vi "CreateGraphMenu_InAreaButNotCurve.vi"(4 "isFloatXY":T1, 6 "isShowYvalue":T1, 9 "Language":refnum<vi>, 11 "菜单输入":refnum<k9>) -> ()   [LabVIEW 2015]
uses:
  Ctrls/YesOrNo.ctl
  GlobalVariables.vi
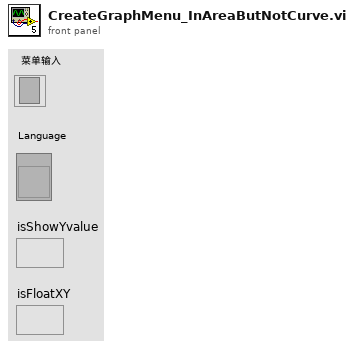
[diagram p1: front panel]
types:
  T1 = typedef "YesOrNo.ctl" = bool
  T2 = cluster{"MenuNames":string[], "MenuTags":string[]}
  T3 = cluster{"Visible":bool, "Color":u32, "LineWidth":u8}
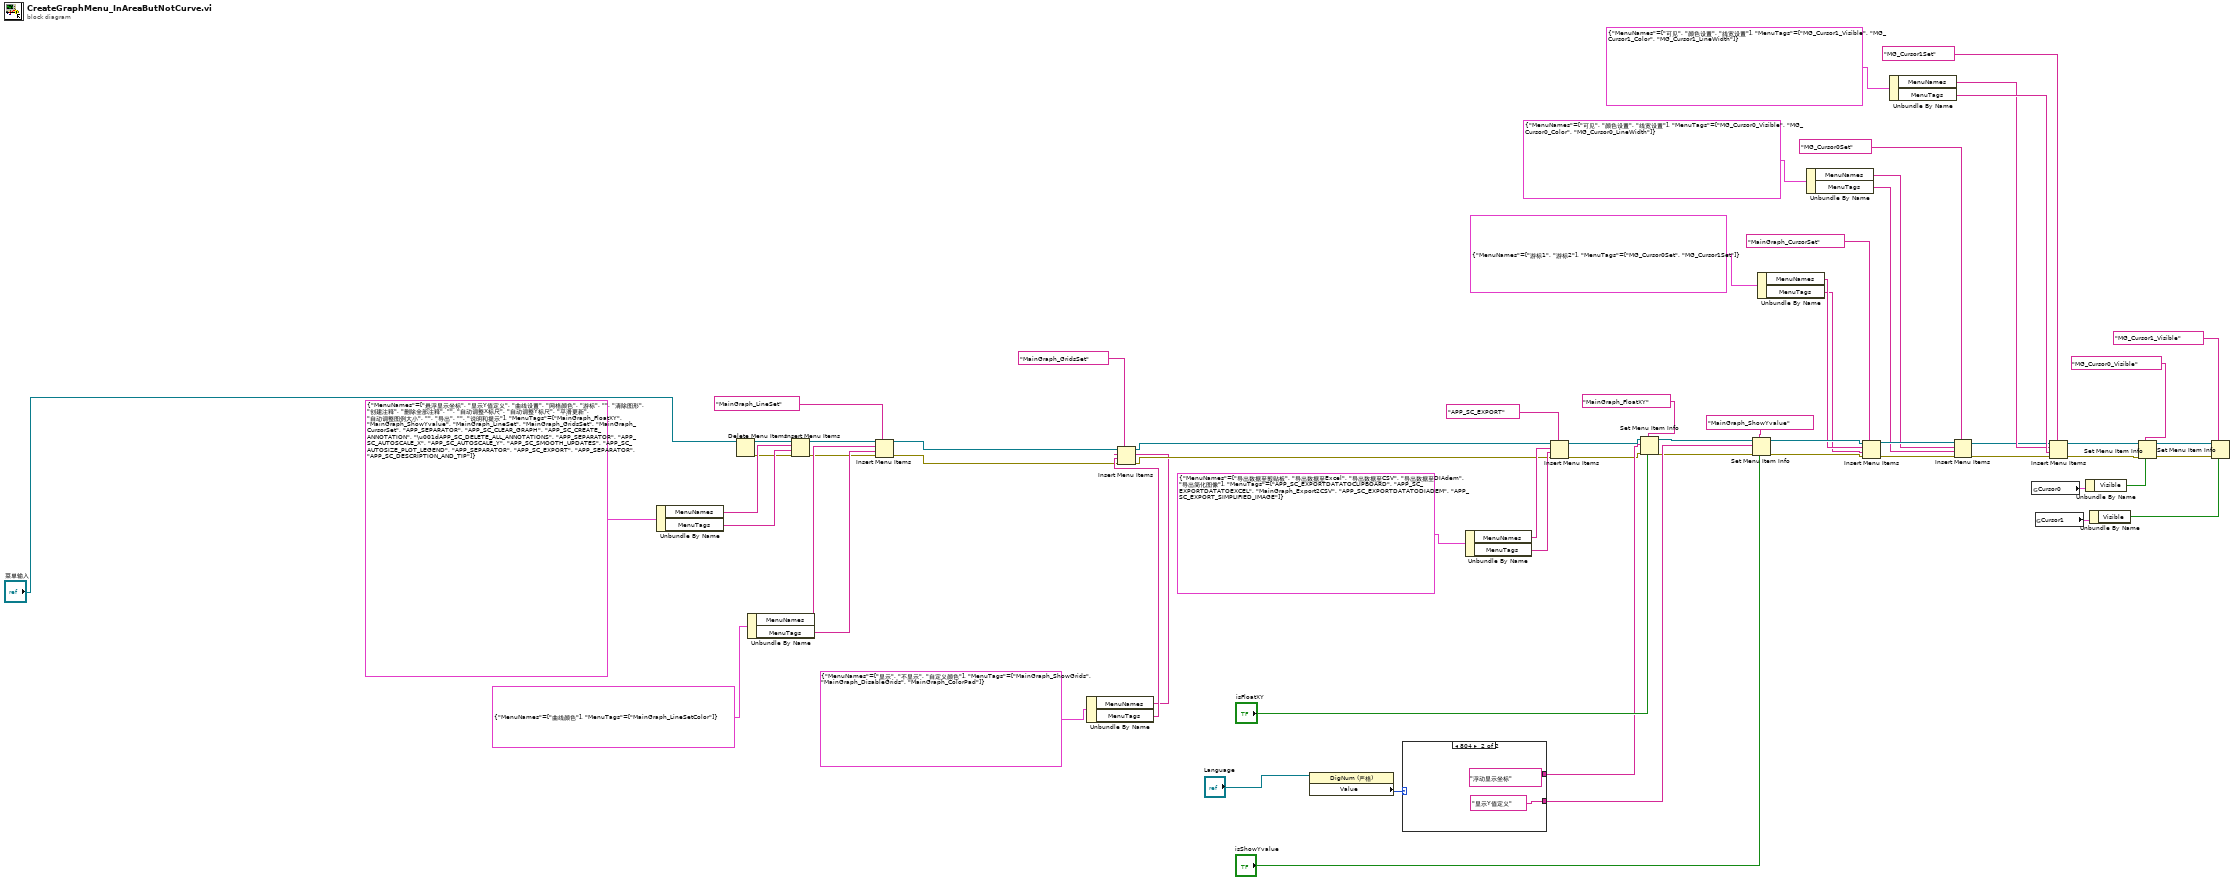
[diagram p0: block diagram]
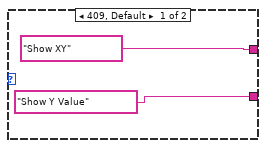
[diagram p2: hidden frame]
diagram:
  n1 = Unbundle By Name(T2 {"MenuNames"=["悬浮显示坐标", "显示Y值定义", "曲线设置", "网格颜色", "游标", "", "清除图形", "创建注释", "删除全部注释", "", "自动调整X标尺", "自动调整Y标尺", "平滑更新", "自动调整图例大小", "", "导出", "", "说明和提示"], "MenuTags"=["MainGraph_FloatXY", "MainGraph_ShowYvalue", "MainGraph_LineSet", "MainGraph_GridsSet", "MainGraph_CursorSet", "APP_SEPARATOR", "APP_SC_CLEAR_GRAPH", "APP_SC_CREATE_ANNOTATION", "\u001dAPP_SC_DELETE_ALL_ANNOTATIONS", "APP_SEPARATOR", "APP_SC_AUTOSCALE_X", "APP_SC_AUTOSCALE_Y", "APP_SC_SMOOTH_UPDATES", "APP_SC_AUTOSIZE_PLOT_LEGEND", "APP_SEPARATOR", "APP_SC_EXPORT", "APP_SEPARATOR", "APP_SC_DESCRIPTION_AND_TIP"]}) -> ("MenuNames"=w50:string[], "MenuTags"=w51:string[])
  n2 = Delete Menu Items(9:"菜单输入") -> (0:w43:errorcluster, 3:w45:refnum<k9>)  [unwired: 3 in]
  n3 = Unbundle By Name(T2 {"MenuNames"=["曲线颜色"], "MenuTags"=["MainGraph_LineSetColor"]}) -> ("MenuNames"=w54:string[], "MenuTags"=w53:string[])
  n4 = Insert Menu Items(6:w43, 7:w51, 8:w50, 9:w45) -> (0:w44:errorcluster, 3:w48:refnum<k9>)  [unwired: 2 in, 1 out]
  n5 = Insert Menu Items(5:"MainGraph_LineSet" ("L10n_menu tag"), 6:w44, 7:w53, 8:w54, 9:w48) -> (0:w29:errorcluster, 3:w30:refnum<k9>)  [unwired: 1 in, 1 out]
  n6 = Unbundle By Name(T2 {"MenuNames"=["显示", "不显示", "自定义颜色"], "MenuTags"=["MainGraph_ShowGrids", "MainGraph_DisableGrids", "MainGraph_ColorPad"]}) -> ("MenuNames"=w56:string[], "MenuTags"=w57:string[])
  n7 = Insert Menu Items(5:"MainGraph_GridsSet" ("L10n_menu tag"), 6:w29, 7:w57, 8:w56, 9:w30) -> (0:w59:errorcluster, 3:w60:refnum<k9>)  [unwired: 1 in, 1 out]
  n8 = property class="DigNum (严格)"(reference="Language") -> ("Value"=w35:u32)  [unwired: 1 in, 2 out]
  n9 = case shown="804" w35 {
    tunnel: ["Show XY" "浮动显示坐标"] -> w39
    tunnel: ["Show Y Value" "显示Y值定义"] -> w40
    frame 409, Default {
    }
    frame 804 {
    }
  }
  n10 = Unbundle By Name(T2 {"MenuNames"=["导出数据至剪贴板", "导出数据至Excel", "导出数据至CSV", "导出数据至DIAdem", "导出简化图像"], "MenuTags"=["APP_SC_EXPORTDATATOCLIPBOARD", "APP_SC_EXPORTDATATOEXCEL", "MainGraph_Export2CSV", "APP_SC_EXPORTDATATODIADEM", "APP_SC_EXPORT_SIMPLIFIED_IMAGE"]}) -> ("MenuNames"=w62:string[], "MenuTags"=w63:string[])
  n11 = Insert Menu Items(5:"APP_SC_EXPORT" ("L10n_menu tag"), 6:w59, 7:w63, 8:w62, 9:w60) -> (0:w33:errorcluster, 3:w34:refnum<k9>)  [unwired: 1 in, 1 out]
  n12 = Set Menu Item Info(6:"isFloatXY", 7:"MainGraph_FloatXY", 8:w33, 10:w39, 11:w34) -> (0:w32:errorcluster)  [unwired: 2 in, 1 out]
  n13 = Set Menu Item Info(6:"isShowYvalue", 7:"MainGraph_ShowYvalue", 8:w32, 10:w40, 11:w34) -> (0:w27:errorcluster, 3:w28:refnum<k9>)  [unwired: 2 in]
  n14 = Unbundle By Name(T2 {"MenuNames"=["游标1", "游标2"], "MenuTags"=["MG_Cursor0Set", "MG_Cursor1Set"]}) -> ("MenuNames"=w25:string[], "MenuTags"=w24:string[])
  n15 = Unbundle By Name(T2 {"MenuNames"=["可见", "颜色设置", "线宽设置"], "MenuTags"=["MG_Cursor0_Visible", "MG_Cursor0_Color", "MG_Cursor0_LineWidth"]}) -> ("MenuNames"=w19:string[], "MenuTags"=w18:string[])
  n16 = Insert Menu Items(5:"MainGraph_CursorSet", 6:w27, 7:w24, 8:w25, 9:w28) -> (0:w21:errorcluster, 3:w22:refnum<k9>)  [unwired: 1 in, 1 out]
  n17 = Unbundle By Name(T2 {"MenuNames"=["可见", "颜色设置", "线宽设置"], "MenuTags"=["MG_Cursor1_Visible", "MG_Cursor1_Color", "MG_Cursor1_LineWidth"]}) -> ("MenuNames"=w14:string[], "MenuTags"=w15:string[])
  n18 = Insert Menu Items(5:"MG_Cursor0Set", 6:w21, 7:w18, 8:w19, 9:w22) -> (0:w12:errorcluster, 3:w13:refnum<k9>)  [unwired: 1 in, 1 out]
  n19 = global read "GlobalVariables.vi" "Cursor0"() -> (w8:T3)
  n20 = global read "GlobalVariables.vi" "Cursor1"() -> (w3:T3)
  n21 = Insert Menu Items(5:"MG_Cursor1Set", 6:w12, 7:w15, 8:w14, 9:w13) -> (0:w10:errorcluster, 3:w9:refnum<k9>)  [unwired: 1 in, 1 out]
  n22 = Unbundle By Name(w8) -> ("Visible"=w7:bool)
  n23 = Unbundle By Name(w3) -> ("Visible"=w2:bool)
  n24 = Set Menu Item Info(6:w7, 7:"MG_Cursor0_Visible", 8:w10, 11:w9) -> (0:w4:errorcluster, 3:w5:refnum<k9>)  [unwired: 3 in]
  n25 = Set Menu Item Info(6:w2, 7:"MG_Cursor1_Visible", 8:w4, 11:w5) -> ()  [unwired: 3 in, 2 out]
